vi "create error headers.vi"(10 "custom error reason":string, 11 "headers in":T1) -> (3 "headers out":T1)   [LabVIEW 2016, in "Basic HTTP server.lvclass"]
uses:
  Basic HTTP server.lvclass
  HTTP headers/http header data.ctl
  HTTP headers/http headers.lvlib
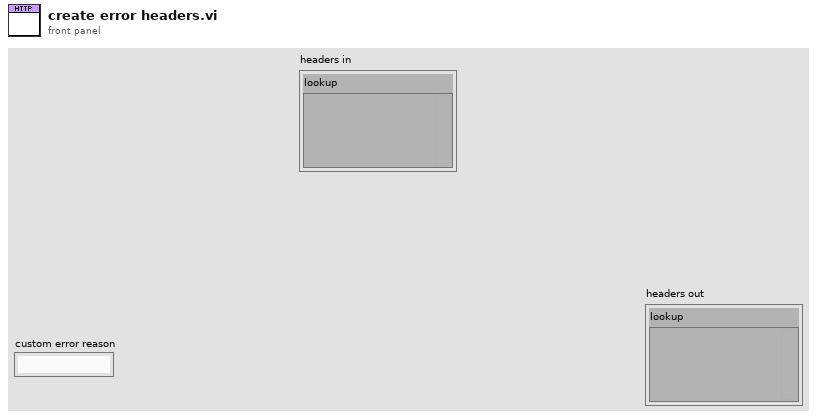
[diagram p1: front panel]
types:
  T1 = typedef "http headers.lvlib/http header data.ctl" = cluster{"lookup":variant}
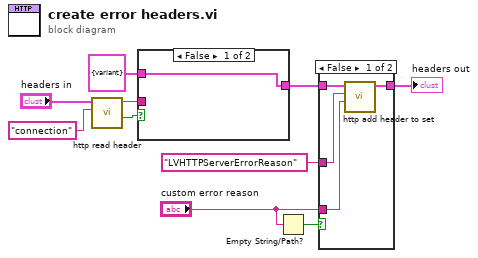
[diagram p0: block diagram]
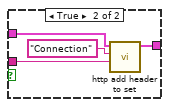
[diagram p3: hidden frame]
diagram:
  n1 = call "http read header.vi"("header field name"="connection" ("name"), "headers"="headers in") -> ("found"=w7:bool, "value"=w1:string)  [unwired: 8 in]
  n2 = case shown="False" w7 {
    tunnel: T1 {"lookup"=variant} ("headers in") -> [w11 w15]
    tunnel: [w11 w14] -> w5
    tunnel: w1 -> [_ w12]
    frame False {
    }
    frame True {
      n3 = call "http add header to set.vi"("header field data"=w12, "header field name"="Connection", "headers in"=w15) -> ("headers out"=w14:T1)  [unwired: 8 in]
    }
  }
  n4 = Empty String/Path?(string/path="custom error reason") -> (empty?=w4:bool)
  n5 = case shown="False" w4 {
    tunnel: [w19 w20] -> w10
    tunnel: w5 -> [w18 w20]
    tunnel: "LVHTTPServerErrorReason" ("error header") -> [w17 _]
    tunnel: "custom error reason" -> [w16 _]
    frame False {
      n6 = call "http add header to set.vi"("header field data"=w16, "header field name"=w17, "headers in"=w18) -> ("headers out"=w19:T1)  [unwired: 8 in]
    }
    frame True {
    }
  }
  "headers out" <- w10
